vi "ConvertTo(arrayDBL).vi"(8 "error in":errorcluster, 9 "Message Payload":variant) -> (0 "error out":errorcluster, 1 "Message Payload DBL Numeric":dbl[](array[numeric]))   [LabVIEW 2017]
doc: "Convert variant to DBL scalar\n\nBolder Software LLC"
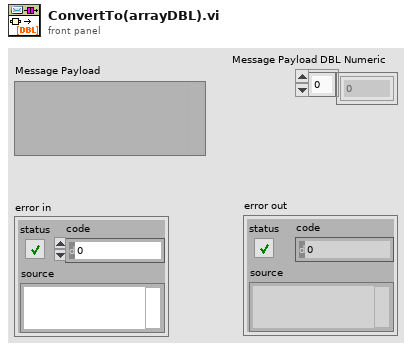
[diagram p1: front panel]
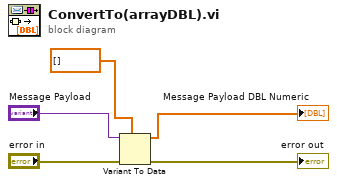
[diagram p0: block diagram]
diagram:
  n1 = Variant To Data(error in="error in", type=dbl[] [], Variant="Message Payload") -> (data=→"Message Payload DBL Numeric":dbl[], error out=→"error out":errorcluster)
